vi "Radoslaw_Wolnik_3.4_12.vi"() -> ()   [LabVIEW 2012]
panel:
  in  "Określ ilość elementów ciągu fibonacciego":i32
  out "Ciąg fibonacciego do określonego powyżej elementu":string
  # "Program oblicza ciąg Fibonacciego od elementu 1 do określonego przez użytkownika poniżej"
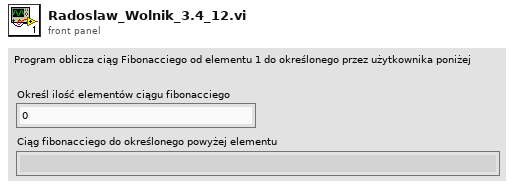
[diagram p1: front panel]
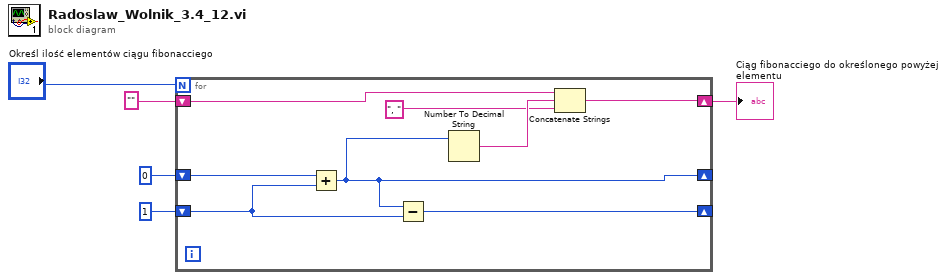
[diagram p0: block diagram]
diagram:
  n1 = for {
    N: "Określ ilość elementów ciągu fibonacciego" -> [_]
    shift-right: [w13] -> _
    shift-left: 1 -> [w10]
    shift-right: [w6] -> _
    shift-left: 0 -> [w9]
    shift-right: [w11] -> w2
    shift-left: "" -> [w12]
    n2 = Add(x=w9, y=w10) -> (x+y=w6:i32)
    n3 = Subtract(x=w6, y=w10) -> (x-y=w13:i32)
    n4 = Number To Decimal String(number=w6) -> (decimal integer string=w8:string)  [unwired: 1 in]
    n5 = Concatenate Strings(w12, w8, ", ") -> (w11:string)
  }
  "Ciąg fibonacciego do określonego powyżej elementu" <- w2
